vi "SetupConfigurationExampleMikrotronCamera.vi"   [LabVIEW 2015]
uses:
  Main/GlobalVariables.vi
types:
  T1 = typedef "CameraInterface.ctl" = cluster{"Close":T2, "Get/Set generic config":T3, "Grab":T4, "Show Settings Dialog":T5, "AdjustBeadPos":T6, "Save/load camera settings":T7}
  T2 = typedef "CICloseType.ctl" = refnum<vi>
  T3 = typedef "CIGetSetGenericConfig.ctl" = refnum<vi>
  T4 = typedef "CIGrabType.ctl" = refnum<vi>
  T5 = typedef "CISettingsDlg.ctl" = refnum<vi>
  T6 = typedef "CIAdjustBeadPos.ctl" = refnum<vi>
  T7 = typedef "CISaveLoadSettings.ctl" = refnum<vi>
  T8 = typedef "CameraInstance.ctl" = cluster{"VI refs":T1, "Camera state":variant}
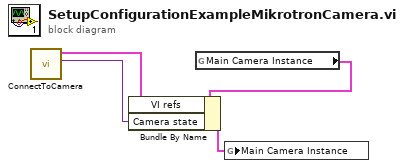
[diagram p0: block diagram]
diagram:
  n1 = call "ConnectToCamera.vi"() -> ("Camera data (out)"=w2:variant, "Camera interface"=w3:T1)  [unwired: 10 in]
  n2 = global read "GlobalVariables.vi" "Main Camera Instance"() -> (w4:T8)
  n3 = Bundle By Name(cluster=w4, "VI refs"=w3, "Camera state"=w2) -> (w1:T8)
  n4 = global write "GlobalVariables.vi" "Main Camera Instance"(w1) -> ()
